vi "SetCursor.vi"(8 "error in (no error)":errorcluster, 10 "icon":u16(ring), 11 "VMUI in":refnum<class "VMUI.lvclass">) -> (0 "error out":errorcluster, 3 "VMUI out":refnum<class "VMUI.lvclass">)   [LabVIEW 2013, in "VMUI.lvclass"]
uses:
  VMUI.lvclass
  <vilib>/Utility/cursorutil.llb/Set Cursor (Icon Pict).vi
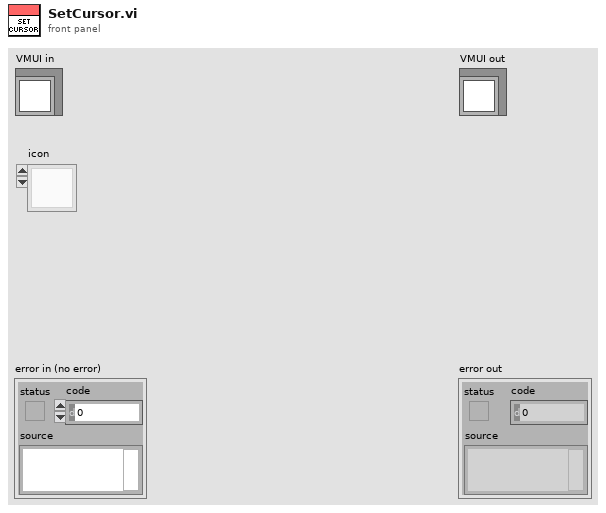
[diagram p1: front panel]
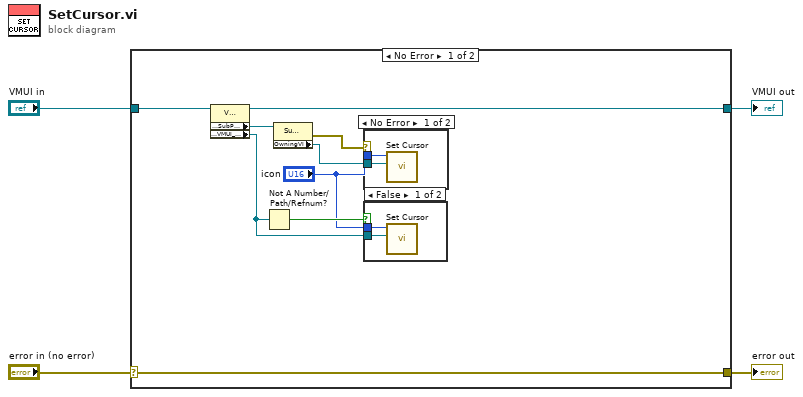
[diagram p0: block diagram]
diagram:
  n1 = case shown="No Error" "error in (no error)" {
    selector: "error in (no error)" -> [w13 w19]
    tunnel: [w13 w19] -> w3
    tunnel: [w10 w18] -> w1
    tunnel: "VMUI in" -> [w11 w18]
    frame No Error {
      n2 = property class="VMUI.lvclass"(reference=w11) -> (reference out=w10:refnum<class "VMUI.lvclass">, "Accessors:SubPanelRef"=w12:refnum<vi>, "Accessors:VMUI_VI_Ref"=w6:refnum<vi>)  [unwired: 1 in, 1 out]
      n3 = Not A Number/Path/Refnum?(number/path/refnum=w6) -> (NaN/Path/Refnum?=w7:bool)
      n4 = property class="SubPnl"(reference=w12) -> (error out=w9:errorcluster, "OwningVI"=w8:refnum<vi>)  [unwired: 1 in, 1 out]
      n5 = case shown="No Error" w9 {
        tunnel: w8 -> [w17 _]
        tunnel: "icon" -> [w16 _]
        frame No Error {
          n6 = call-poly <vilib>:"Set Cursor.vi"("VI reference (current VI)"=w17, "icon"=w16) -> ()  [unwired: 8 in, 2 out]
        }
        frame Error {
        }
      }
      n7 = case shown="False" w7 {
        tunnel: w6 -> [w15 _]
        tunnel: "icon" -> [w14 _]
        frame False {
          n8 = call-poly <vilib>:"Set Cursor.vi"("VI reference (current VI)"=w15, "icon"=w14) -> ()  [unwired: 8 in, 2 out]
        }
        frame True {
        }
      }
    }
    frame Error {
    }
  }
  "error out" <- w3
  "VMUI out" <- w1
